vi "ROI grp-Show or hide group ROIs.vi"(8 "error in (no error)":errorcluster, 10 "Visible?":bool=TRUE) -> (0 "error out":errorcluster)   [LabVIEW 2020]
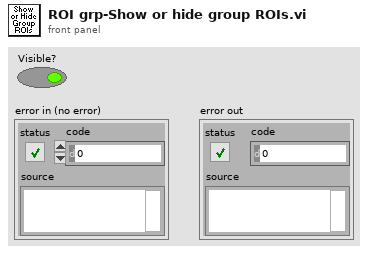
[diagram p1: front panel]
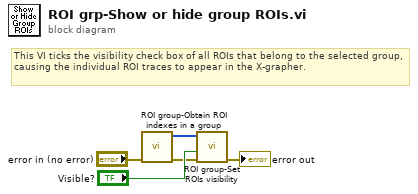
[diagram p0: block diagram]
diagram:
  # "This VI ticks the visibility check box of all ROIs that belong to the selected group, causing the individual ROI traces to appear in the X-grapher."
  n1 = call "ROI group-Obtain ROI indexes in a group.vi"("error in (no error)"="error in (no error)") -> ("error out"=w2:errorcluster, "Group's ROIs indexes"=w3:i32[])  [unwired: 9 in]
  n2 = call "ROI group-Set ROIs visibility.vi"("error in (no error)"=w2, "Visible?"="Visible?", "Indexes of new ROIs to make visible"=w3) -> ("error out"=→"error out":errorcluster)  [unwired: 8 in]
